vi "VOUT.vi"(8 "error in (no error)":errorcluster, 10 "Channel":T1, 11 "refnum in":T2) -> (0 "error out":errorcluster, 1 "Vout?":dbl, 2 "sVout":string, 3 "refnum out":T2, 4 "question out":string)   [LabVIEW 2020, in "Korad KA3305P.lvlib"]
uses:
  Korad KA3305P.lvlib
  Reference.ctl
  Channels.ctl
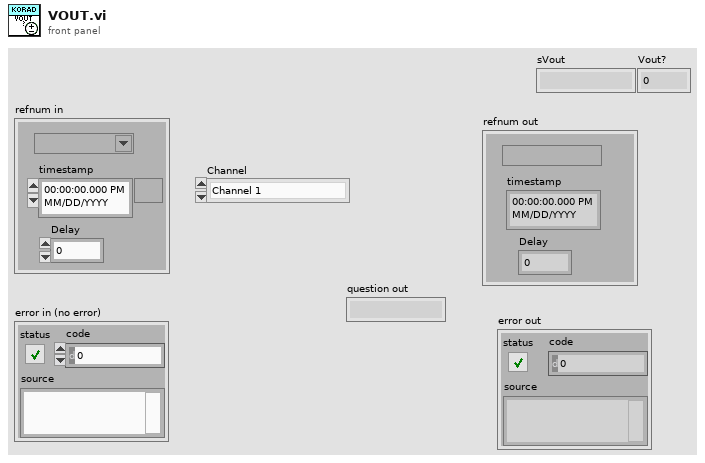
[diagram p1: front panel]
types:
  T1 = typedef "Korad KA3305P.lvlib/Channels.ctl" = enum16{"Channel 1", "Channel 2"}
  T2 = typedef "Korad KA3305P.lvlib/Reference.ctl" = cluster{"refnum":refnum<visa-resource-name>, "timestamp":timestamp, "Delay":dbl}
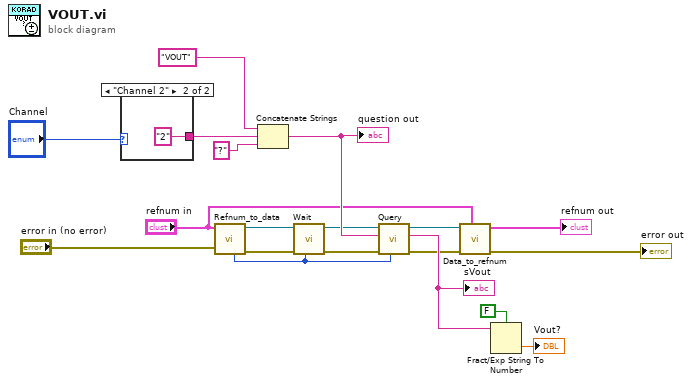
[diagram p0: block diagram]
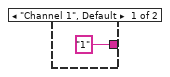
[diagram p2: hidden frame]
diagram:
  n1 = case shown="\"Channel 2\"" "Channel" {
    tunnel: ["1" "2"] -> w3
    frame "Channel 1", Default {
    }
    frame "Channel 2" {
    }
  }
  n2 = call "Refnum_to_data.vi"("error in (no error)"="error in (no error)", "refnum in"="refnum in") -> ("error out"=w6:errorcluster, "DAQ refnum out"=w7:refnum<visa-resource-name>, "delay out"=w16:u32)  [unwired: 7 in]
  n3 = Concatenate Strings("VOUT" ("string"), w3, "?" ("string")) -> (w13:string)
  "question out" <- w13
  n4 = call "Wait.vi"("milliseconds to wait"=w16, "error in (no error)"=w6, "refnum in"=w7) -> ("error out"=w12:errorcluster, "refnum out"=w11:refnum<visa-resource-name>)  [unwired: 7 in]
  n5 = call "Query.vi"("delay (55ms)"=w16, "error in (no error)"=w12, "data in"=w13, "refnum in"=w11) -> ("error out"=w15:errorcluster, "data out"=w17:string, "refnum out"=w14:refnum<visa-resource-name>)  [unwired: 5 in]
  "sVout" <- w17
  n6 = call "Data_to_refnum.vi"("refnum in"="refnum in", "error in (no error)"=w15, "DAQ refnum in"=w14) -> ("error out"=→"error out":errorcluster, "refnum out"=→"refnum out":T2)  [unwired: 7 in]
  n7 = Fract/Exp String To Number(use system decimal point (T)=FALSE, string=w17) -> (number=→"Vout?":dbl)  [unwired: 2 in, 1 out]
